vi "Scanner Action-Status Move Single.vi"(8 "error in (no error)":errorcluster, 10 "Message Data":variant, 11 "Data Cluster in":T1={"Link"={"Connection"=enum."USB", "Host or IP address (TCP/IP)"="", "Port (Serial/USB)"="COM1"}, "VISA resource"="", "Writer Queue"=refnum, "Status"=FALSE}) -> (0 "error out":errorcluster, 3 "Data Cluster out":T1={"Link"={"Connection"=enum."USB", "Host or IP address (TCP/IP)"="", "Port (Serial/USB)"="COM1"}, "VISA resource"="", "Writer Queue"=refnum, "Status"=FALSE})   [LabVIEW 2020, in "Hiden Scanner.lvlib"]
uses:
  Hiden Scanner.lvlib
  support/Message Queue/Message Cluster.ctl
  support/Message Queue/Message Queue.lvlib
  support/HW Message Cluster.ctl
  Scanner Hardware Configuration.ctl
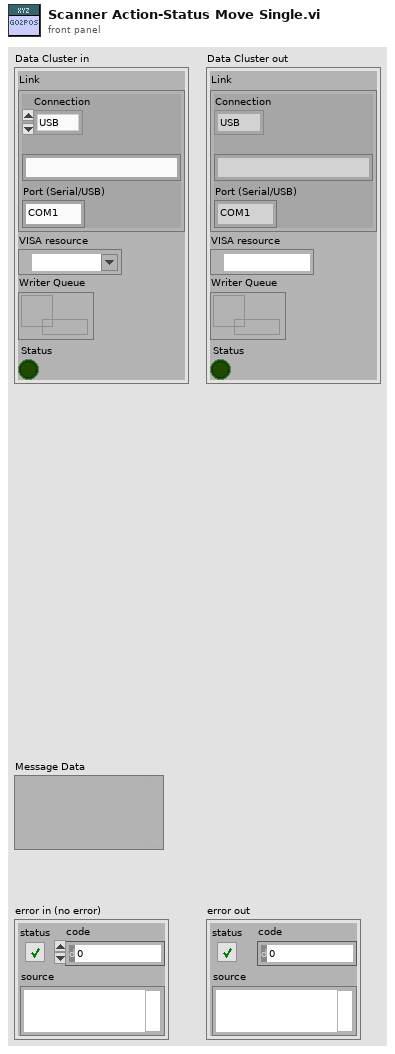
[diagram p1: front panel]
types:
  T1 = typedef "Hiden Scanner.lvlib/Scanner Hardware Configuration.ctl" = cluster{"Link":cluster{"Connection":enum16{"Serial", "TCP/IP", "USB"}, "Host or IP address (TCP/IP)":string, "Port (Serial/USB)":string}, "VISA resource":refnum<visa-resource-name>, "Writer Queue":refnum<queue>, "Status":bool}
  T2 = cluster{"Axis":enum16{"X", "Y", "Z", "A"}, "dValue":dbl}
  T3 = typedef "Message Queue.lvlib/HW Message Cluster.ctl" = cluster{"Writer Queue":refnum<queue>, "Writer Data":T4}
  T4 = typedef "Message Queue.lvlib/Message Cluster.ctl" = cluster{"Message":string, "Message Data":variant}
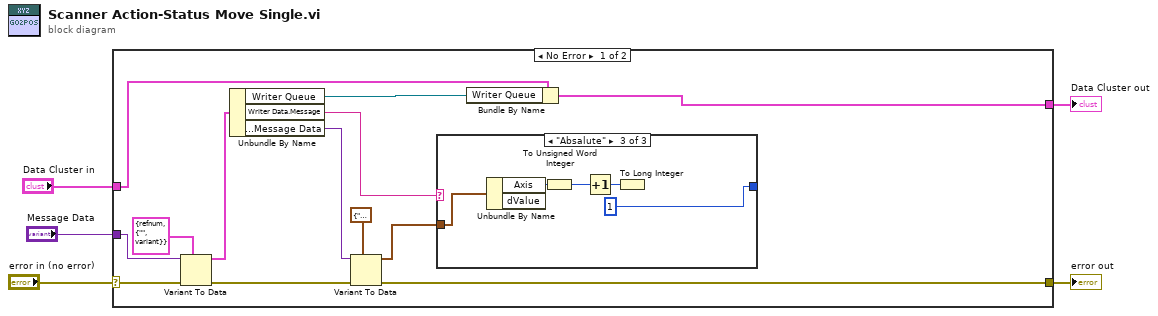
[diagram p0: block diagram]
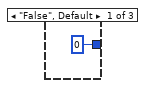
[diagram p2: hidden frame]
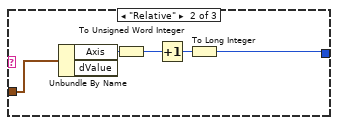
[diagram p3: hidden frame]
diagram:
  n1 = case shown="No Error" "error in (no error)" {
    selector: "error in (no error)" -> [w11 w30]
    tunnel: "Message Data" -> [w10 _]
    tunnel: [w9 w31] -> w4
    tunnel: "Data Cluster in" -> [w12 w31]
    tunnel: [w18 w30] -> w2
    frame No Error {
      n2 = Variant To Data(error in=w11, type=T3 {"Writer Queue"=refnum, "Writer Data"={"Message"="", "Message Data"=variant}}, Variant=w10) -> (data=w13:T3, error out=w15:errorcluster)
      n3 = Unbundle By Name(w13) -> ("Writer Queue"=w16:refnum<queue>, "Writer Data.Message"=w8:string, "Writer Data.Message Data"=w14:variant)
      n4 = Variant To Data(error in=w15, type=T2 {"Axis"=enum."X", "dValue"=0.0}, Variant=w14) -> (data=w6:T2, error out=w18:errorcluster)
      n5 = case shown="\"Absalute\"" w8 {
        tunnel: w6 -> [_ w24 w29]
        tunnel: [0 ("function return") w20 1 ("bWait")] -> _
        frame "False", Default {
        }
        frame "Relative" {
          n6 = Unbundle By Name(w24) -> ("Axis"=w23:enum16{"X", "Y", "Z", "A"})  [unwired: 1 out]
          n7 = To Unsigned Word Integer(number=w23) -> (unsigned 16bit integer=w22:u16)
          n8 = Increment(x=w22) -> (x+1=w21:u16)
          n9 = To Long Integer(number=w21) -> (32bit integer=w20:i32)
        }
        frame "Absalute" {
          n10 = Unbundle By Name(w29) -> ("Axis"=w28:enum16{"X", "Y", "Z", "A"})  [unwired: 1 out]
          n11 = To Unsigned Word Integer(number=w28) -> (unsigned 16bit integer=w27:u16)
          n12 = Increment(x=w27) -> (x+1=w26:u16)
          n13 = To Long Integer(number=w26) -> ()  [unwired: 1 out]
        }
      }
      n14 = Bundle By Name(cluster=w12, "Writer Queue"=w16) -> (w9:T1)
    }
    frame Error {
    }
  }
  "Data Cluster out" <- w4
  "error out" <- w2
